vi "calculate current exp time.vi"(8 "error in (no error)":errorcluster, 11 "CCDCamera in":refnum<class "Simulated Camera.lvclass">) -> (0 "error out":errorcluster, 3 "CCDCamera out":refnum<class "Simulated Camera.lvclass">)   [LabVIEW 2018, in "Simulated Camera.lvclass"]
doc: "Calculate the exposure time of the current acquisition\n\nThis calculation is based on the timestamp get after the star of the acquisition"
uses:
  Simulated Camera.lvclass
  Simulated Camera.lvclass/Simulated Camera.ctl
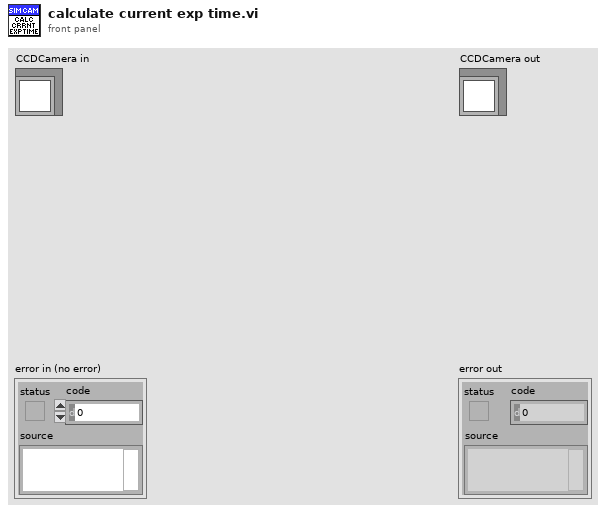
[diagram p1: front panel]
types:
  T1 = cluster{"FRAMES_DONE":u16, "CCD_STATUS":string, "CURRENT_TEMPERATURE":i16, "TEMPERATURE_STATUS":string, "FRAME_EXPOSURE_TIME":sgl, "SERIAL_NUMBER":u16, "ACQUIRING":bool, "POWER":bool}
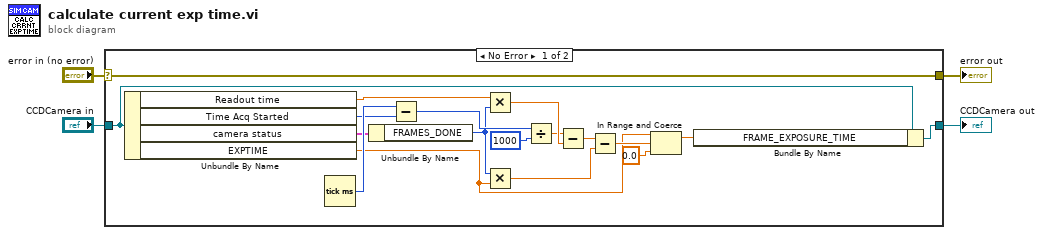
[diagram p0: block diagram]
diagram:
  n1 = case shown="No Error" "error in (no error)" {
    selector: "error in (no error)" -> [w22 w24]
    tunnel: [w22 w24] -> w2
    tunnel: [w5 w23] -> w1
    tunnel: "CCDCamera in" -> [w6 w23]
    frame No Error {
      n2 = Unbundle By Name(w6) -> ("Readout time"=w11:dbl, "Time Acq Started"=w20:u32, "camera status"=w17:T1, "EXPTIME"=w7:dbl)
      n3 = Tick Count (ms)() -> (millisecond timer value=w21:u32)
      n4 = Unbundle By Name(w17) -> ("FRAMES_DONE"=w12:u16)
      n5 = Subtract(x=w21, y=w20) -> (x-y=w19:u32)
      n6 = Multiply(x=w11, y=w12) -> (x*y=w10:dbl)
      n7 = Multiply(x=w12, y=w7) -> (x*y=w13:dbl)
      n8 = Divide(x=w19, y=1000) -> (x/y=w9:dbl)
      n9 = Subtract(x=w9, y=w10) -> (x-y=w8:dbl)
      n10 = Subtract(x=w8, y=w13) -> (x-y=w15:dbl)
      n11 = In Range and Coerce(upper limit=w7, x=w15, lower limit=sgl 0.0) -> (coerced(x)=w14:dbl)  [unwired: 1 out]
      n12 = Bundle By Name(cluster=w6, "FRAME_EXPOSURE_TIME"=w14) -> (w5:refnum<class "Simulated Camera.lvclass">)
    }
    frame Error {
    }
  }
  "error out" <- w2
  "CCDCamera out" <- w1
